vi "toml_find_section.vi"(10 "section":string[](array[string]), 11 "sections":T1[](array[typedef])) -> (3 "index":i32)   [LabVIEW 2017]
uses:
  toml_fg_section.ctl
  toml_fg_row.ctl
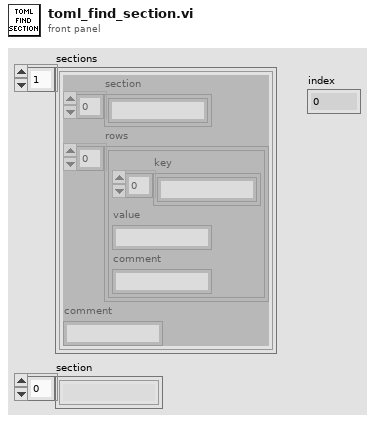
[diagram p1: front panel]
types:
  T1 = typedef "toml_fg_section.ctl" = cluster{"section":string[], "rows":T2[], "comment":string}
  T2 = typedef "toml_fg_row.ctl" = cluster{"key":string[], "value":string, "comment":string}
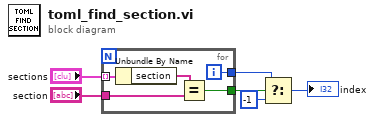
[diagram p0: block diagram]
diagram:
  n1 = for {
    tunnel: "sections" -> [w11] mode=indexing
    tunnel: "section" -> [w9]
    tunnel: [w8] -> w4
    tunnel: [w7] -> w3
    i -> [w8]
    n2 = Unbundle By Name(w11) -> ("section"=w10:string[])
    n3 = Equal?(x=w10, y=w9) -> (x = y?=w7:bool)
  }
  n4 = Select(t=w4, s=w3, f=-1) -> (s? t:f=→"index":i32)
